vi "Pico2000 - AdcToVolts.vi"(9 "Max ADC":i16, 10 "Range Index":u16, 11 "Data (Volts)":dbl) -> (3 "Data (ADC counts)":i16)   [LabVIEW 2017]
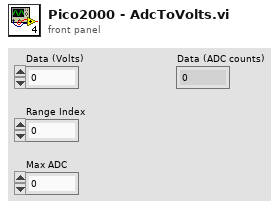
[diagram p1: front panel]
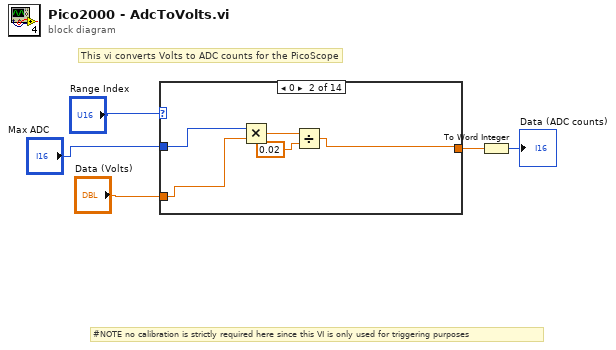
[diagram p0: block diagram]
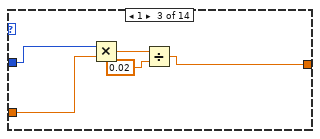
[diagram p3: hidden frame]
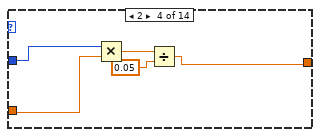
[diagram p4: hidden frame]
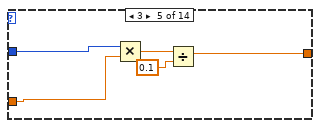
[diagram p5: hidden frame]
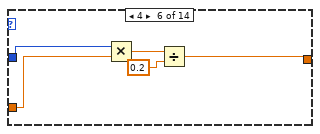
[diagram p6: hidden frame]
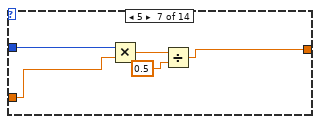
[diagram p7: hidden frame]
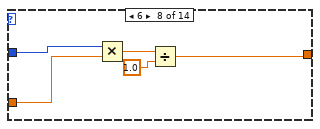
[diagram p8: hidden frame]
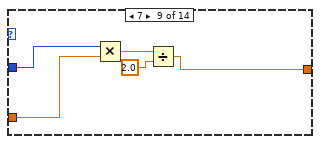
[diagram p9: hidden frame]
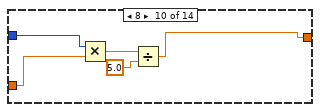
[diagram p10: hidden frame]
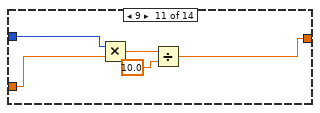
[diagram p11: hidden frame]
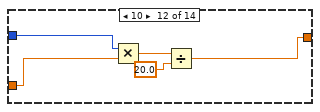
[diagram p12: hidden frame]
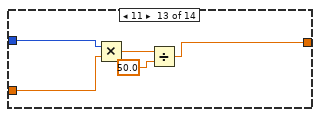
[diagram p13: hidden frame]
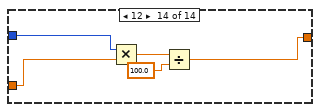
[diagram p14: hidden frame]
diagram:
  # "#NOTE no calibration is strictly required here since this VI is only used for triggering purposes"
  # "This vi converts Volts to ADC counts for the PicoScope"
  n1 = case shown="0" "Range Index" {
    tunnel: [w6 w7 w14 w17 w24 w27 w32 w39 w44 w47 w52 w57 w62 w69] -> w2
    tunnel: "Data (Volts)" -> [w6 w8 w15 w18 w22 w29 w33 w37 w42 w48 w53 w58 w63 w67]
    tunnel: "Max ADC" -> [_ w9 w13 w19 w23 w28 w34 w38 w43 w49 w54 w59 w64 w68]
    frame Default {
    }
    frame 0 {
      n2 = Multiply(x=w9, y=w8) -> (x*y=w11:dbl)
      n3 = Divide(x=w11, y=0.02 ("x")) -> (x/y=w7:dbl)
    }
    frame 1 {
      n4 = Multiply(x=w13, y=w15) -> (x*y=w16:dbl)
      n5 = Divide(x=w16, y=0.02 ("x")) -> (x/y=w14:dbl)
    }
    frame 2 {
      n6 = Multiply(x=w19, y=w18) -> (x*y=w21:dbl)
      n7 = Divide(x=w21, y=0.05 ("x")) -> (x/y=w17:dbl)
    }
    frame 3 {
      n8 = Multiply(x=w23, y=w22) -> (x*y=w25:dbl)
      n9 = Divide(x=w25, y=0.1 ("x")) -> (x/y=w24:dbl)
    }
    frame 4 {
      n10 = Multiply(x=w28, y=w29) -> (x*y=w30:dbl)
      n11 = Divide(x=w30, y=0.2 ("x")) -> (x/y=w27:dbl)
    }
    frame 5 {
      n12 = Multiply(x=w34, y=w33) -> (x*y=w35:dbl)
      n13 = Divide(x=w35, y=0.5 ("x")) -> (x/y=w32:dbl)
    }
    frame 6 {
      n14 = Multiply(x=w38, y=w37) -> (x*y=w40:dbl)
      n15 = Divide(x=w40, y=1.0 ("x")) -> (x/y=w39:dbl)
    }
    frame 7 {
      n16 = Multiply(x=w43, y=w42) -> (x*y=w45:dbl)
      n17 = Divide(x=w45, y=2.0 ("x")) -> (x/y=w44:dbl)
    }
    frame 8 {
      n18 = Multiply(x=w49, y=w48) -> (x*y=w50:dbl)
      n19 = Divide(x=w50, y=5.0 ("x")) -> (x/y=w47:dbl)
    }
    frame 9 {
      n20 = Multiply(x=w54, y=w53) -> (x*y=w55:dbl)
      n21 = Divide(x=w55, y=10.0 ("x")) -> (x/y=w52:dbl)
    }
    frame 10 {
      n22 = Multiply(x=w59, y=w58) -> (x*y=w60:dbl)
      n23 = Divide(x=w60, y=20.0 ("x")) -> (x/y=w57:dbl)
    }
    frame 11 {
      n24 = Multiply(x=w64, y=w63) -> (x*y=w65:dbl)
      n25 = Divide(x=w65, y=50.0 ("x")) -> (x/y=w62:dbl)
    }
    frame 12 {
      n26 = Multiply(x=w68, y=w67) -> (x*y=w70:dbl)
      n27 = Divide(x=w70, y=100.0 ("x")) -> (x/y=w69:dbl)
    }
  }
  n28 = To Word Integer(number=w2) -> (16bit integer=→"Data (ADC counts)":i16)
